vi "Path name select.vi"(1 "In":string) -> (0 "Out":string)   [LabVIEW 2013]
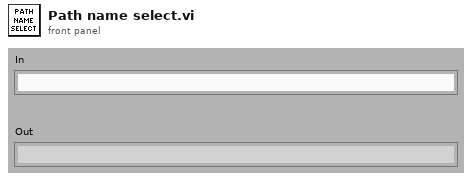
[diagram p1: front panel]
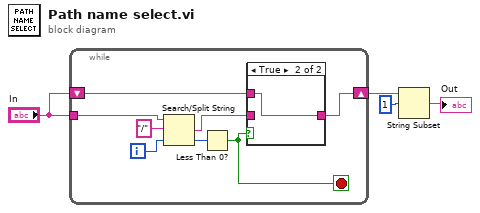
[diagram p0: block diagram]
diagram:
  n1 = while {
    shift-right: [w11] -> w3
    shift-left: "In" -> [w7]
    tunnel: "In" -> [w5]
    i -> [w6]
    stop <- w12 stop-if-true
    n2 = Search/Split String(string=w5, search string/char (-)="/" ("regular expression"), offset (0)=w6) -> (match + rest of string=w9:string, offset of match=w10:i32)  [unwired: 1 out]
    n3 = Less Than 0?(x=w10) -> (x < 0?=w12:bool)
    n4 = case shown="True" w12 {
      tunnel: w9 -> [w13 _]
      tunnel: [w13 w14] -> w11
      tunnel: w7 -> [_ w14]
      frame False {
      }
      frame True {
      }
    }
  }
  n5 = String Subset(string=w3, offset (0)=1) -> (substring=→"Out":string)  [unwired: 1 in]
